vi "NewConnection.vi"(8 "error in (no error)":errorcluster, 10 "Connection Information":T1, 11 "Connections Controller in":refnum<class "Connections Controller.lvclass">) -> (0 "error out":errorcluster, 3 "Connections Controller out":refnum<class "Connections Controller.lvclass">)   [LabVIEW 2023, in "TCP_Listener.lvlib" / "Connections Controller.lvclass"]
uses:
  Connections Controller.lvclass
  TypeDefinitions/ConnectionInformation.ctl
  TCP_Listener.lvlib
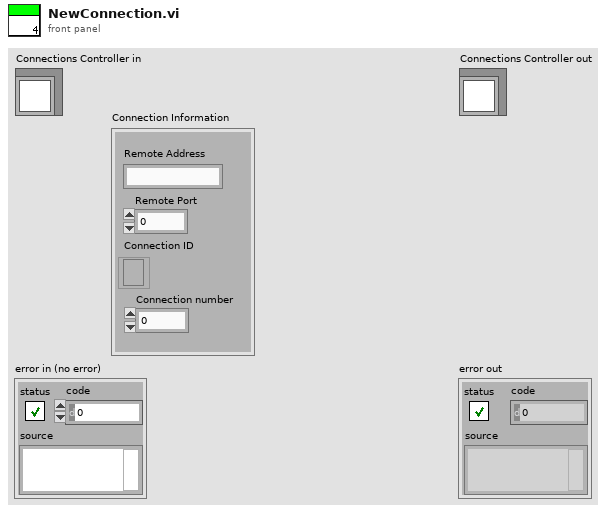
[diagram p1: front panel]
types:
  T1 = typedef "TCP_Listener.lvlib/ConnectionInformation.ctl" = cluster{"Remote Address":string, "Remote Port":u16, "Connection ID":refnum<k5>, "Connection number":dbl}
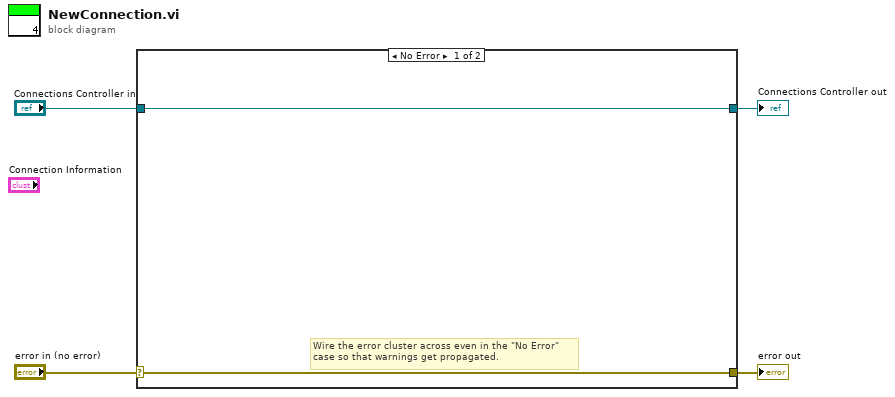
[diagram p0: block diagram]
diagram:
  n1 = case shown="No Error" "error in (no error)" {
    selector: "error in (no error)" -> [w5 w8]
    tunnel: [w5 w8] -> w3
    tunnel: [w6 w7] -> w1
    tunnel: "Connections Controller in" -> [w6 w7]
    frame No Error {
      # "Wire the error cluster across even in the \"No Error\"\ncase so that warnings get propagated."
    }
    frame Error {
    }
  }
  "error out" <- w3
  "Connections Controller out" <- w1
